vi "PID_PressureCtl_Screenshots.vi"(8 "error in":errorcluster, 11 "Screenshots Pfad":path) -> (0 "error out 2":errorcluster caption="error out", 3 "Screenshots Pfad  2":path caption="Screenshots Pfad")   [LabVIEW 2020, in "Backup.lvlib"]
uses:
  Backup.lvlib
  Seiten/Erweiterte Konfig/PID-Parameter Druckregler einstellen v2.vi
  Seiten/Erweiterte Konfig/Erweiterte Konfig.lvlib
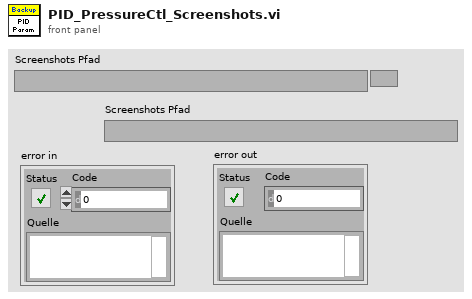
[diagram p1: front panel]
types:
  T1 = enum32{"Bad", "Idle", "Run top level", "Running"}
  T2 = typedef "imagedata.ctl" = cluster{"image type":i32, "image depth":i32, "image":u8[], "mask":u8[], "colors":u32[], "Rectangle":cluster{"left":i16, "top":i16, "right":i16, "bottom":i16}}
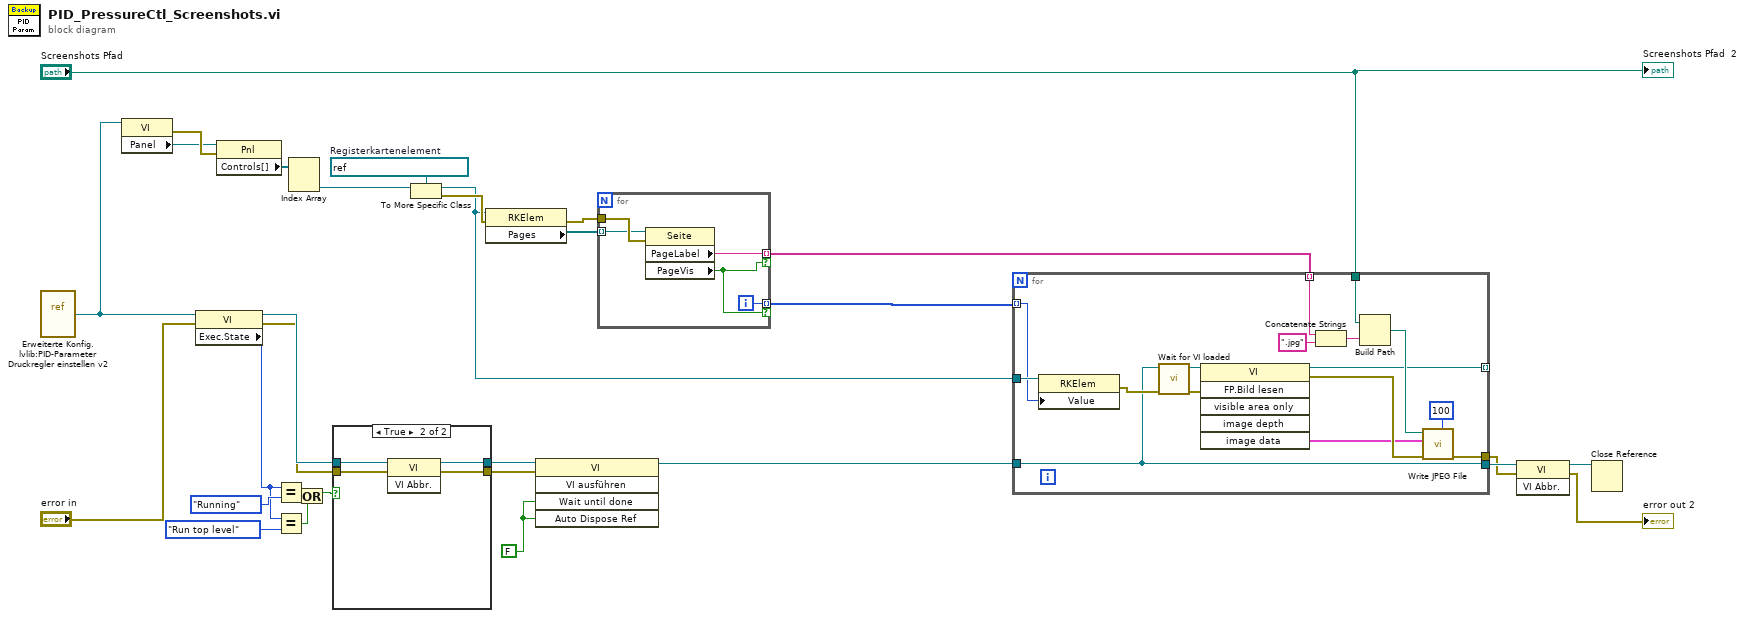
[diagram p0: block diagram]
diagram:
  w15 = refnum<vi> refnum  # Registerkartenelement
  w28 = FALSE
  n1 = vi-ref "Erweiterte Konfig.lvlib:PID-Parameter Druckregler einstellen v2.vi"() -> (w2:refnum<vi>)
  n2 = property class="VI"(reference=w2) -> (error out=w18:errorcluster, "Panel"=w17:refnum<vi>)  [unwired: 1 in, 1 out]
  n3 = property class="VI"(reference=w2, error in="error in") -> (reference out=w27:refnum<vi>, error out=w24:errorcluster, "Exec.State"=w21:T1)
  n4 = property class="Pnl"(reference=w17, error in=w18) -> ("Controls[]"=w16:refnum<vi>[])  [unwired: 2 out]
  n5 = Equal?(x=w21, y=T1."Running" ("Ausführung:Status")) -> (x = y?=w25:bool)
  n6 = Equal?(x=w21, y=T1."Run top level" ("Ausführung:Status")) -> (x = y?=w19:bool)
  n7 = Index Array(array=w16) -> (element #2=w12:refnum<vi>)  [unwired: 2 in, 1 out]
  n8 = Or(x=w25, y=w19) -> (x .or. y?=w20:bool)
  n9 = case shown="True" w20 {
    tunnel: w27 -> [w32 w36]
    tunnel: [w32 w35] -> w26
    tunnel: w24 -> [w31 w34]
    tunnel: [w31 w33] -> w23
    frame False {
    }
    frame True {
      n10 = invoke class="VI" method="VI Abbr."(reference=w36, error in=w34) -> (reference out=w35:refnum<vi>, error out=w33:errorcluster)  [unwired: 1 in, 1 out]
    }
  }
  n11 = To More Specific Class(target class=w15, reference=w12) -> (specific class reference=w9:refnum<vi>, error out=w14:errorcluster)  [unwired: 1 in]
  n12 = property class="RKElem"(reference=w9, error in=w14) -> (error out=w13:errorcluster, "Pages"=w11:refnum<vi>[])  [unwired: 1 out]
  n13 = invoke class="VI" method="VI ausführen"(reference=w26, error in=w23, "Wait until done"=w28, "Auto Dispose Ref"=w28) -> (reference out=w1:refnum<vi>)  [unwired: 1 in, 4 out]
  n14 = for {
    tunnel: w13 -> [w41]
    tunnel: w11 -> [w40] mode=indexing
    tunnel: [w39] -> w10 mode=indexing if=w37
    tunnel: [w38] -> w3 mode=indexing if=w37
    i -> [w38]
    n15 = property class="Seite"(reference=w40, error in=w41) -> ("PageLabel"=w39:string, "PageVis"=w37:bool)  [unwired: 2 out]
  }
  n16 = for {
    tunnel: [w49] -> _ mode=indexing
    tunnel: w10 -> [w48] mode=indexing
    tunnel: [w47] -> w6
    tunnel: w9 -> [w46]
    tunnel: w1 -> [w44]
    tunnel: [w44] -> w7
    tunnel: "Screenshots Pfad" -> [w43]
    tunnel: w3 -> [w42] mode=indexing
    n17 = property class="RKElem"(reference=w46, "Value"=w42) -> (error out=w45:errorcluster)  [unwired: 1 in, 1 out]
    n18 = call "Wait for VI loaded.vi"("error in"=w45, "VI Referenz"=w44) -> ("error out"=w57:errorcluster, "VI Referenz out"=w56:refnum<vi>)  [unwired: 7 in, 1 out]
    n19 = invoke class="VI" method="FP.Bild lesen"(reference=w56, error in=w57) -> (reference out=w49:refnum<vi>, error out=w51:errorcluster, "image data"=w50:T2)  [unwired: 4 in, 3 out]
    n20 = Concatenate Strings(w48, ".jpg" ("String")) -> (w54:string)
    n21 = Build Path(base path=w43, name or relative path=w54) -> (appended path=w53:path)
    n22 = call <vilib>:"Write JPEG File.vi"("quality (80)"=100, "error in (no error)"=w51, "image data"=w50, "path to JPEG file"=w53) -> ("error out"=w47:errorcluster)  [unwired: 6 in, 1 out]
  }
  n23 = invoke class="VI" method="VI Abbr."(reference=w7, error in=w6) -> (reference out=w8:refnum<vi>, error out=→"error out 2":errorcluster)  [unwired: 1 in, 1 out]
  n24 = Close Reference(reference=w8) -> ()  [unwired: 1 in, 1 out]
  "Screenshots Pfad  2" <- "Screenshots Pfad"
